vi "FGA Add Service to Component.vi"(1 "ServiceRec":T1, 2 "Component Id":u8, 3 "Node Id":u8) -> (0 "Added?":bool)   [LabVIEW 2009]
uses:
  ServiceRec.ctl
  cRIO/Functional Global Variables/Actions for FG's.ctl
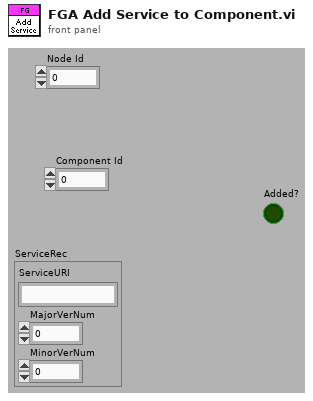
[diagram p1: front panel]
types:
  T1 = typedef "ServiceRec.ctl" = cluster{"ServiceURI":string, "MajorVerNum":u8, "MinorVerNum":u8}
  T2 = typedef "NodeRec.ctl" = cluster{"Node Id":u8, "ComponentSeq":T3[]}
  T3 = typedef "ComponentRec.ctl" = cluster{"Component Id":u8, "Instance Id":u8, "ServiceSeq":T1[]}
  T4 = typedef "Actions for FG's.ctl" = enum16{"Read", "Write"}
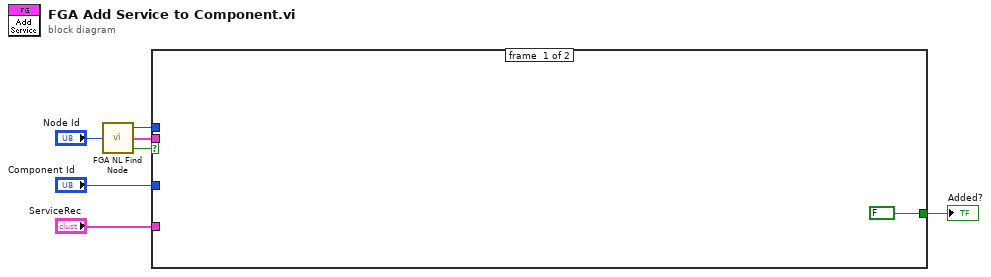
[diagram p0: block diagram]
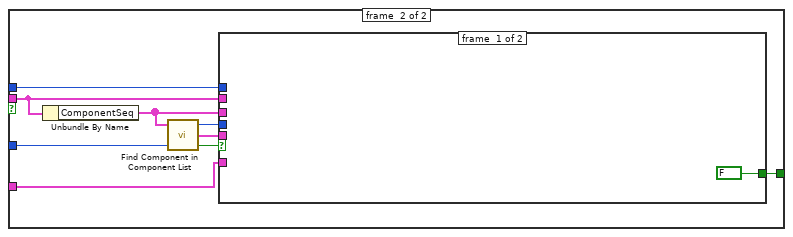
[diagram p2: hidden frame]
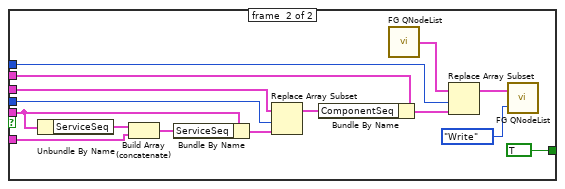
[diagram p3: hidden frame]
diagram:
  n1 = call "FGA NL Find Node.vi"("Node ID"="Node Id") -> ("Record Exists?"=w4:bool, "NodeRec"=w6:T2, "Node Index"=w2:i32)  [unwired: 2 in]
  n2 = case shown="True" w4 {
    tunnel: w6 -> [_ w13]
    tunnel: "Component Id" -> [_ w17]
    tunnel: "ServiceRec" -> [_ w15]
    tunnel: w2 -> [_ w10]
    tunnel: [FALSE ("Added?") w9] -> w1
    frame #0 {
    }
    frame #1 {
      n3 = Unbundle By Name(w13) -> ("ComponentSeq"=w12:T3[])
      n4 = call "Find Component in Component List.vi"("Component Id"=w17, "ComponentSeq"=w12) -> ("Record Exists?"=w16:bool, "ComponentRec"=w14:T3, "Component Index"=w11:i32)  [unwired: 1 in]
      n5 = case shown="True" w16 {
        tunnel: w15 -> [_ w32]
        tunnel: w14 -> [_ w31]
        tunnel: w13 -> [_ w29]
        tunnel: w12 -> [_ w28]
        tunnel: w11 -> [_ w26]
        tunnel: w10 -> [_ w23]
        tunnel: [FALSE ("Added?") TRUE ("Added?")] -> w9
        frame #0 {
        }
        frame #1 {
          n6 = Unbundle By Name(w31) -> ("ServiceSeq"=w33:T1[])
          n7 = Build Array (concatenate)(w33, w32) -> (w30:T1[])
          n8 = Bundle By Name(cluster=w31, "ServiceSeq"=w30) -> (w27:T3)
          n9 = Replace Array Subset(array=w28, new element=w27, index=w26) -> (w25:T3[])
          n10 = Bundle By Name(cluster=w29, "ComponentSeq"=w25) -> (w22:T2)
          n11 = call "FG QNodeList.vi"() -> ("NodeList out"=w24:T2[])  [unwired: 2 in]
          n12 = Replace Array Subset(array=w24, new element=w22, index=w23) -> (w20:T2[])
          n13 = call "FG QNodeList.vi"("FG Action (Read)"=Actions_for_FG's."Write", "NodeList in"=w20) -> ()  [unwired: 1 out]
        }
      }
    }
  }
  "Added?" <- w1
